vi "仪器参数设置.vi"(11 "仪器参数":T1) -> (2 "仪器参数 2":T1, 3 "check？":bool)   [LabVIEW 2016, in "斯坦道总磷.lvlib"]
uses:
  <vilib>/Utility/miscctls.llb/LVPointTypeDef.ctl
  <vilib>/addons/database/Auxilliary.llb/DB Tools DataTypes.ctl
  <vilib>/regexp/Match Regular Expression.xnode
  <vilib>/addons/database/NI_Database_API.lvlib
panel:
  in  "仪器参数表":i32(listbox)
  in  "取消":bool
  in  "确定":bool
  # "仪器参数"
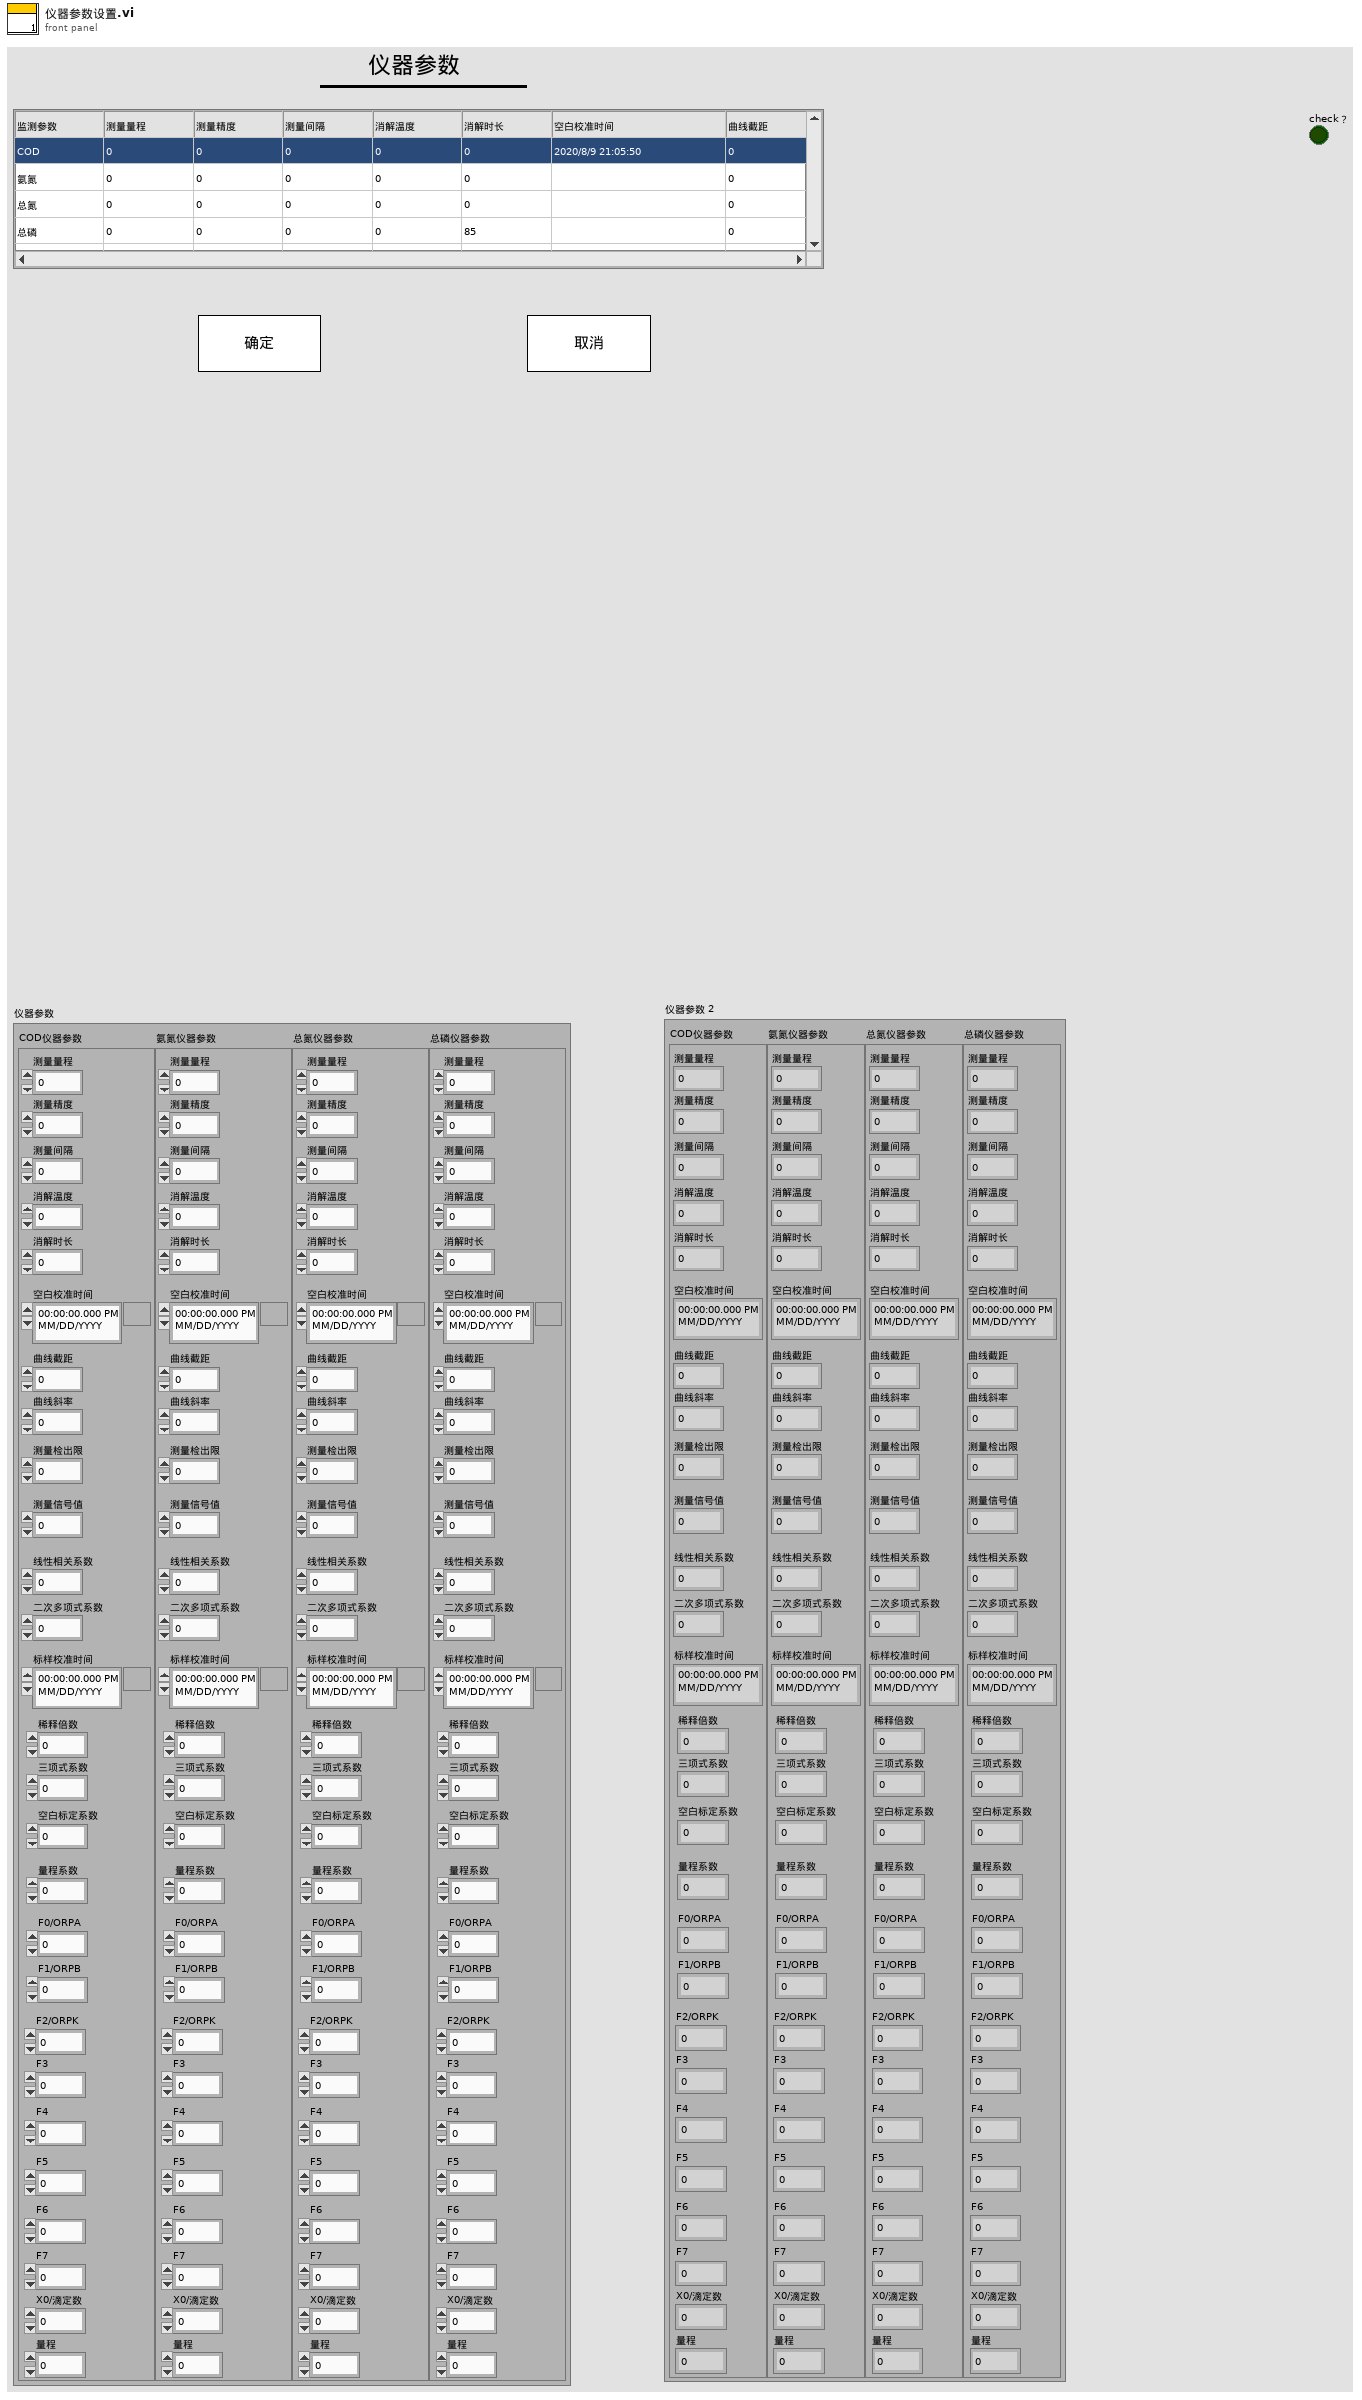
[diagram p1: front panel]
types:
  T1 = cluster{"COD仪器参数":cluster{"测量量程":dbl, "测量精度":dbl, "测量间隔":dbl, "消解温度":dbl, "消解时长":dbl, "空白校准时间":timestamp, "曲线截距":dbl, "曲线斜率":dbl, "测量检出限":dbl, "测量信号值":dbl, "线性相关系数":dbl, "二次多项式系数":dbl, "标样校准时间":timestamp, "稀释倍数":dbl, "三项式系数":dbl, "空白标定系数":dbl, "量程系数":dbl, "F0/ORPA":dbl, "F1/ORPB":dbl, "F2/ORPK":dbl, "F3":dbl, "F4":dbl, "F5":dbl, "F6":dbl, "F7":dbl, "X0/滴定数":dbl, "量程":dbl}, "氨氮仪器参数":cluster{"测量量程":dbl, "测量精度":dbl, "测量间隔":dbl, "消解温度":dbl, "消解时长":dbl, "空白校准时间":timestamp, "曲线截距":dbl, "曲线斜率":dbl, "测量检出限":dbl, "测量信号值":dbl, "线性相关系数":dbl, "二次多项式系数":dbl, "标样校准时间":timestamp, "稀释倍数":dbl, "三项式系数":dbl, "空白标定系数":dbl, "量程系数":dbl, "F0/ORPA":dbl, "F1/ORPB":dbl, "F2/ORPK":dbl, "F3":dbl, "F4":dbl, "F5":dbl, "F6":dbl, "F7":dbl, "X0/滴定数":dbl, "量程":dbl}, "总氮仪器参数":cluster{"测量量程":dbl, "测量精度":dbl, "测量间隔":dbl, "消解温度":dbl, "消解时长":dbl, "空白校准时间":timestamp, "曲线截距":dbl, "曲线斜率":dbl, "测量检出限":dbl, "测量信号值":dbl, "线性相关系数":dbl, "二次多项式系数":dbl, "标样校准时间":timestamp, "稀释倍数":dbl, "三项式系数":dbl, "空白标定系数":dbl, "量程系数":dbl, "F0/ORPA":dbl, "F1/ORPB":dbl, "F2/ORPK":dbl, "F3":dbl, "F4":dbl, "F5":dbl, "F6":dbl, "F7":dbl, "X0/滴定数":dbl, "量程":dbl}, "总磷仪器参数":cluster{"测量量程":dbl, "测量精度":dbl, "测量间隔":dbl, "消解温度":dbl, "消解时长":dbl, "空白校准时间":timestamp, "曲线截距":dbl, "曲线斜率":dbl, "测量检出限":dbl, "测量信号值":dbl, "线性相关系数":dbl, "二次多项式系数":dbl, "标样校准时间":timestamp, "稀释倍数":dbl, "三项式系数":dbl, "空白标定系数":dbl, "量程系数":dbl, "F0/ORPA":dbl, "F1/ORPB":dbl, "F2/ORPK":dbl, "F3":dbl, "F4":dbl, "F5":dbl, "F6":dbl, "F7":dbl, "X0/滴定数":dbl, "量程":dbl}}
  T2 = typedef "NI_Database_API.lvlib/DB Tools DataTypes.ctl" = enum16{"String", "Long (I32)", "Single (SGL)", "Double (DBL)", "Date/Time", "Binary"}
  T3 = typedef "LVPointTypeDef.ctl" = cluster{"Horizontal":i16, "Vertical":i16}
  T4 = typedef "LVPoint32TypeDef.ctl" = cluster{"Horizontal":i32, "Vertical":i32}
  T5 = typedef "LVRowAndColumnTypeDef.ctl" = cluster{"Row":i32, "Column":i32}
  T6 = cluster{"COD":bool, "氨氮":bool, "总氮":bool, "总磷":bool}
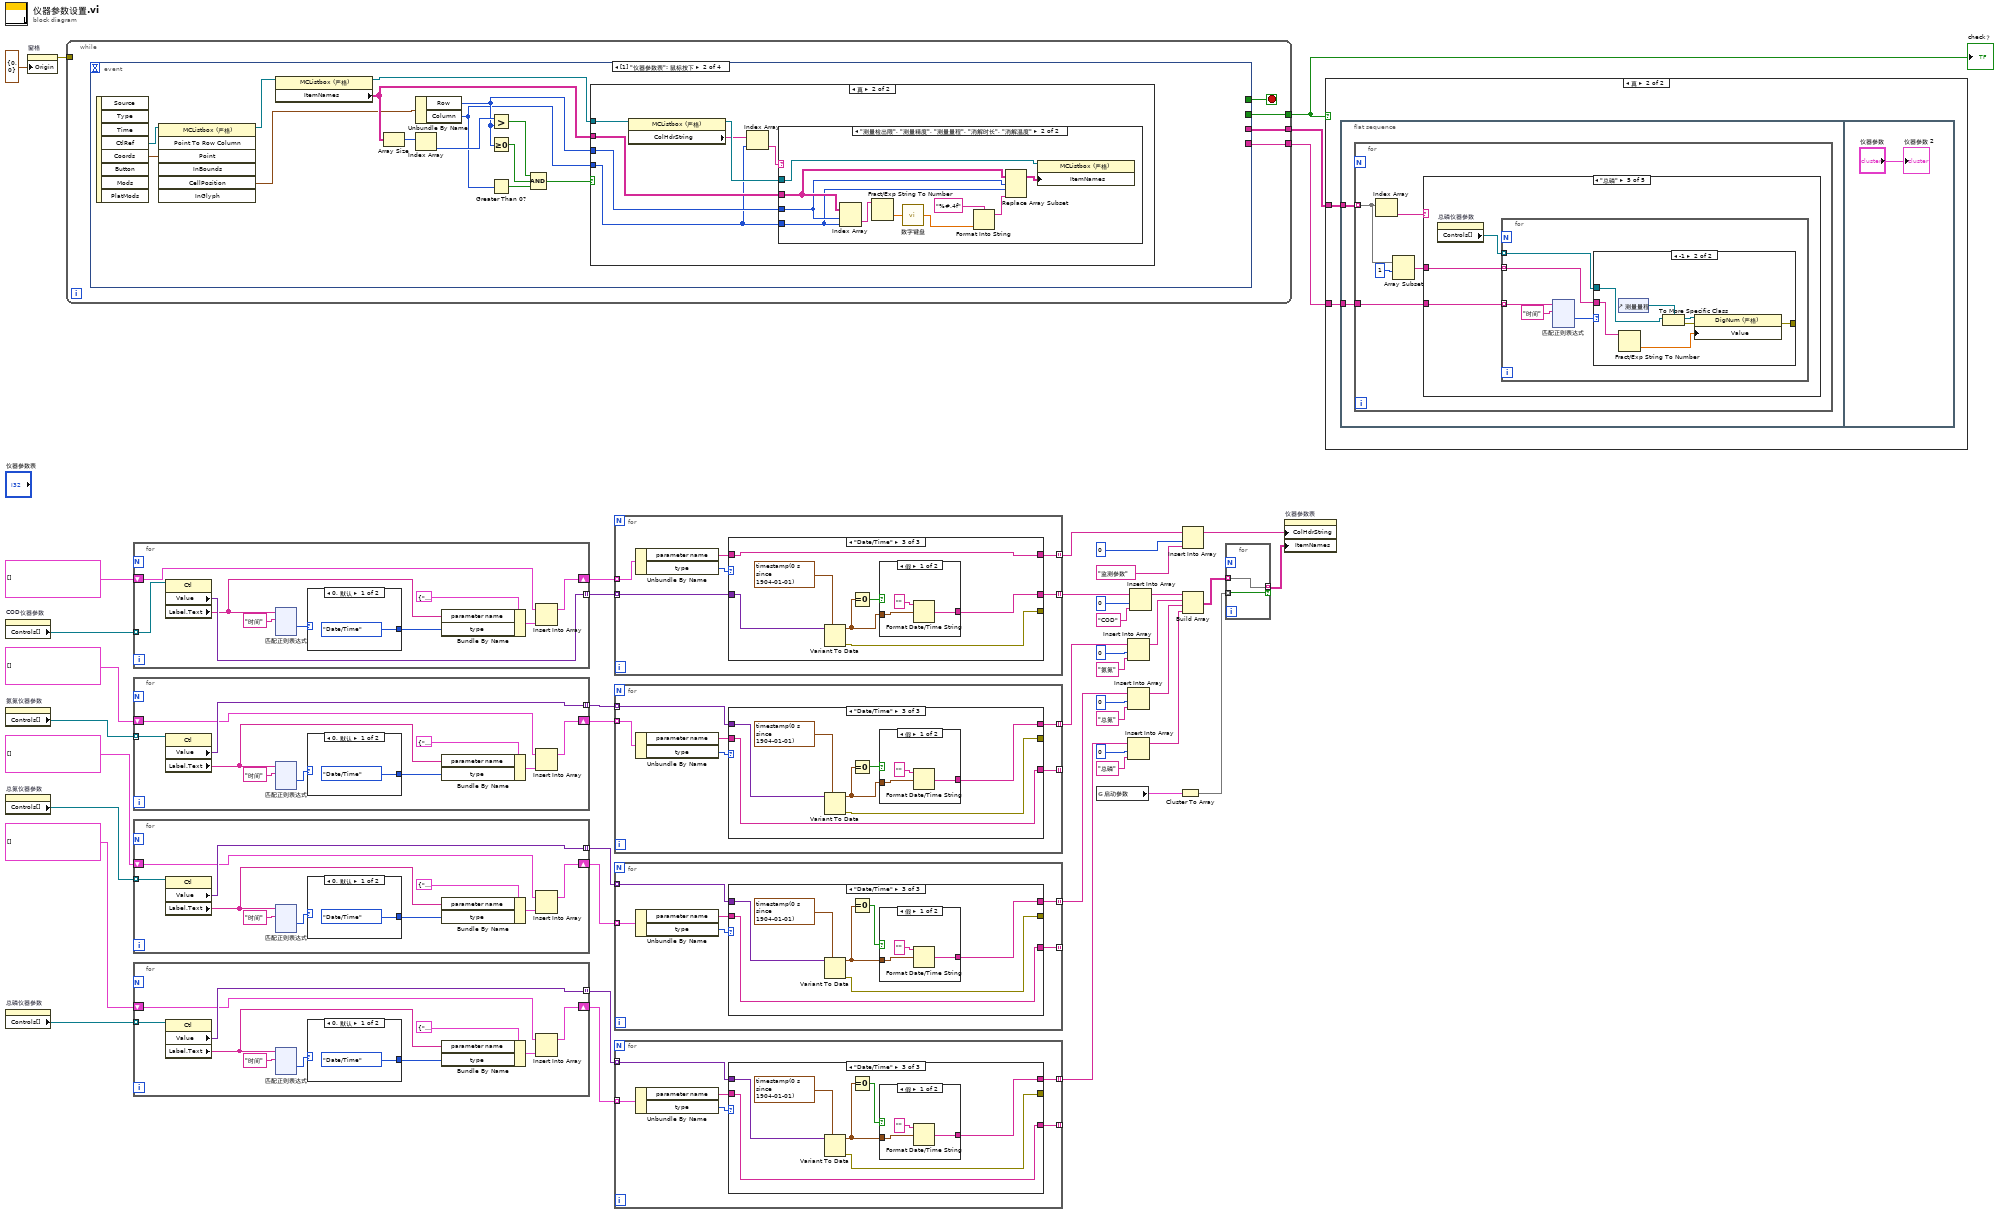
[diagram p0: block diagram]
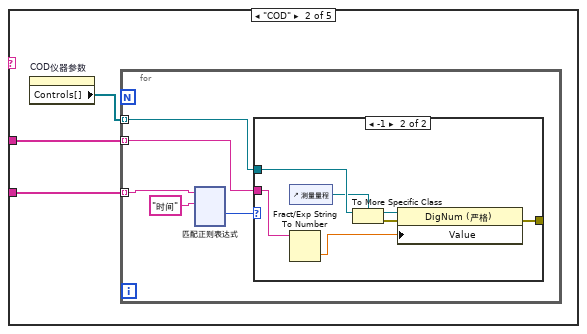
[diagram p4: hidden frame]
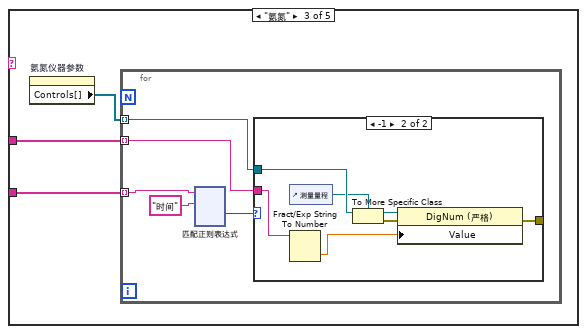
[diagram p6: hidden frame]
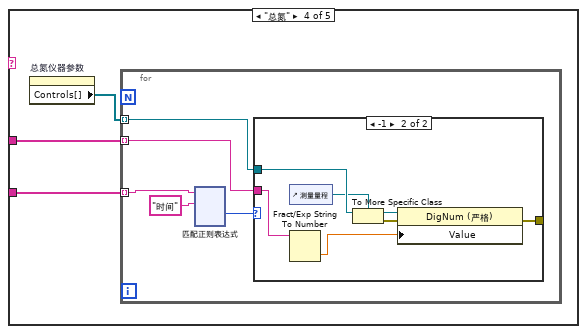
[diagram p8: hidden frame]
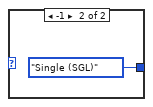
[diagram p11: hidden frame]
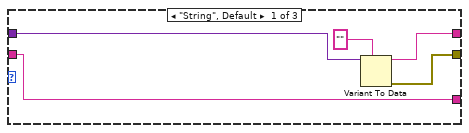
[diagram p12: hidden frame]
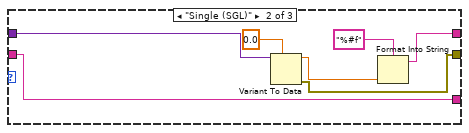
[diagram p13: hidden frame]
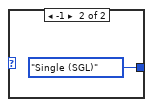
[diagram p15: hidden frame]
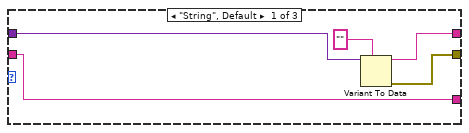
[diagram p16: hidden frame]
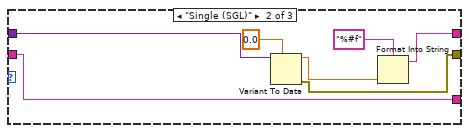
[diagram p17: hidden frame]
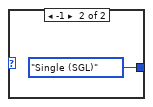
[diagram p19: hidden frame]
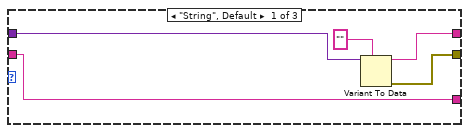
[diagram p20: hidden frame]
diagram:
  n1 = property on="COD仪器参数" class="Clust (严格)"() -> ("Controls[]"=w39:refnum<vi>[])  [unwired: 2 in, 2 out]
  n2 = property on="氨氮仪器参数" class="Clust (严格)"() -> ("Controls[]"=w38:refnum<vi>[])  [unwired: 2 in, 2 out]
  n3 = property on="总氮仪器参数" class="Clust (严格)"() -> ("Controls[]"=w31:refnum<vi>[])  [unwired: 2 in, 2 out]
  n4 = property on="总磷仪器参数" class="Clust (严格)"() -> ("Controls[]"=w30:refnum<vi>[])  [unwired: 2 in, 2 out]
  n5 = property on="窗格" class="Pane"("Origin"=T3 {"Horizontal"=0, "Vertical"=0} ("原点")) -> (error out=w44:errorcluster)  [unwired: 2 in, 1 out]
  n6 = while {
    tunnel: w44 -> [_]
    tunnel: [w48] -> w7
    tunnel: [w47] -> w6
    tunnel: [w46] -> w5
    stop <- w49 stop-if-true
    n7 = event shown="[1] \"仪器参数表\": 鼠标按下" {
      selector: _ -> [_ _ _ _]
      dyn-events: _ -> [_ _ _ _]
      timeout: _ -> [_ _ _ _]
      tunnel: [_ _ TRUE TRUE] -> w49
      tunnel: [_ _ _ "确定"] -> w48
      tunnel: [_ _ _ w83] -> w47
      tunnel: [_ _ _ w82] -> w46
      event Timeout {
        n8 = event-data() -> ()  [unwired: 1 in, 3 out]
      }
      event "仪器参数表": Mouse Down {
        n9 = event-data() -> ("CtlRef"=w63:refnum<vi>, "Coords"=w62:T4)  [unwired: 1 in, 6 out]
        n10 = invoke class="MCListbox (严格)" method="Point To Row Column"(reference=w63, "Point"=w62) -> (reference out=w51:refnum<vi>, "CellPosition"=w50:T5)  [unwired: 5 in, 5 out]
        n11 = property class="MCListbox (严格)"(reference=w51) -> (reference out=w52:refnum<vi>, "ItemNames"=w55:string[][])  [unwired: 1 in, 1 out]
        n12 = Array Size(array=w55) -> (size(s)=w59:i32[])
        n13 = Unbundle By Name(w50) -> ("Row"=w54:i32, "Column"=w53:i32)
        n14 = Index Array(array=w59) -> (element=w58:i32)  [unwired: 1 in]
        n15 = Greater?(x=w58, y=w54) -> (0:w57:bool)
        n16 = Greater Or Equal To 0?(x=w54) -> (x >= 0?=w56:bool)
        n17 = Greater Than 0?(x=w53) -> (x > 0?=w61:bool)
        n18 = Compound Arithmetic op=AND ("复合运算")(w57, w56, w61) -> (w60:bool)
        n19 = case shown="真" w60 {
          tunnel: w55 -> [_ w70]
          tunnel: w54 -> [_ w69]
          tunnel: w53 -> [_ w65]
          tunnel: w52 -> [_ w68]
          frame False {
          }
          frame True {
            n20 = property class="MCListbox (严格)"(reference=w68) -> (reference out=w67:refnum<vi>, "ColHdrString"=w66:string[])  [unwired: 1 in, 1 out]
            n21 = Index Array(array=w66, index=w65) -> (element=w64:string)
            n22 = case shown="\"测量检出限\", \"测量精度\", \"测量量程\", \"消解时长\", \"消解温度\"" w64 {
              tunnel: w70 -> [_ w76]
              tunnel: w69 -> [_ w75]
              tunnel: w65 -> [_ w74]
              tunnel: w67 -> [_ w71]
              frame Default {
              }
              frame "测量检出限", "测量精度", "测量量程", "消解时长", "消解温度" {
                n23 = Index Array(array=w76, index (row)=w75, index (col)=w74) -> (element=w80:string)
                n24 = Fract/Exp String To Number(string=w80) -> (number=w79:dbl)  [unwired: 3 in, 1 out]
                n25 = call "数字键盘.vi"("OldNumber"=w79) -> ("NewNumber"=w78:dbl)
                n26 = Format Into String(format string="%#.4f" ("格式字符串"), w78) -> (resulting string=w73:string)  [unwired: 2 in, 1 out]
                n27 = Replace Array Subset(array=w76, new element=w73, index (row)=w75, index (col)=w74) -> (w72:string[][])
                n28 = property class="MCListbox (严格)"(reference=w71, "ItemNames"=w72) -> ()  [unwired: 1 in, 2 out]
              }
            }
          }
        }
      }
      event "取消": Value Change; Panel Close {
        n29 = event-data() -> ()  [unwired: 1 in, 3 out]
      }
      event "确定": Value Change {
        n30 = event-data() -> ()  [unwired: 1 in, 6 out]
        n31 = property on="仪器参数表" class="MCListbox (严格)"() -> ("ItemNames"=w83:string[][], "ColHdrString"=w82:string[])  [unwired: 2 in, 2 out]
      }
    }
  }
  "check？" <- w7
  n32 = for {
    tunnel: w39 -> [w95] mode=indexing
    tunnel: [w94] -> w43 mode=indexing
    shift-right: [w92] -> w40
    shift-left: cluster{"parameter name":string, "type":T2}[] [] ("parameters out") -> [w93]
    n33 = property class="Ctl"(reference=w95) -> ("Value"=w94:variant, "Label.Text"=w90:string)  [unwired: 1 in, 2 out]
    n34 = xnode "匹配正则表达式"("输入字符串"=w90, "正则表达式"="时间") -> ("匹配后偏移量"=w88:i32)  [unwired: 4 in, 4 out]
    n35 = case shown="0, 默认" w88 {
      tunnel: [DB_Tools_DataTypes."Date/Time" ("type") DB_Tools_DataTypes."Single (SGL)" ("type")] -> w87
      frame 0, Default {
      }
      frame -1 {
      }
    }
    n36 = Bundle By Name(cluster=cluster{"parameter name":string, "type":T2} {"parameter name"="", "type"=enum."String"} ("parameter information"), "parameter name"=w90, "type"=w87) -> (w86:cluster{"parameter name":string, "type":T2})
    n37 = Insert Into Array(array=w93, new element=w86) -> (w92:cluster{"parameter name":string, "type":T2}[])  [unwired: 1 in]
  }
  n38 = for {
    tunnel: w38 -> [w221] mode=indexing
    tunnel: [w220] -> w35 mode=indexing
    shift-right: [w218] -> w37
    shift-left: cluster{"parameter name":string, "type":T2}[] [] ("parameters out") -> [w219]
    n39 = property class="Ctl"(reference=w221) -> ("Value"=w220:variant, "Label.Text"=w216:string)  [unwired: 1 in, 2 out]
    n40 = xnode "匹配正则表达式"("输入字符串"=w216, "正则表达式"="时间") -> ("匹配后偏移量"=w214:i32)  [unwired: 4 in, 4 out]
    n41 = case shown="0, 默认" w214 {
      tunnel: [DB_Tools_DataTypes."Date/Time" ("type") DB_Tools_DataTypes."Single (SGL)" ("type")] -> w213
      frame 0, Default {
      }
      frame -1 {
      }
    }
    n42 = Bundle By Name(cluster=cluster{"parameter name":string, "type":T2} {"parameter name"="", "type"=enum."String"} ("parameter information"), "parameter name"=w216, "type"=w213) -> (w212:cluster{"parameter name":string, "type":T2})
    n43 = Insert Into Array(array=w219, new element=w212) -> (w218:cluster{"parameter name":string, "type":T2}[])  [unwired: 1 in]
  }
  n44 = for {
    tunnel: w31 -> [w347] mode=indexing
    tunnel: [w346] -> w34 mode=indexing
    shift-right: [w344] -> w32
    shift-left: cluster{"parameter name":string, "type":T2}[] [] ("parameters out") -> [w345]
    n45 = property class="Ctl"(reference=w347) -> ("Value"=w346:variant, "Label.Text"=w342:string)  [unwired: 1 in, 2 out]
    n46 = xnode "匹配正则表达式"("输入字符串"=w342, "正则表达式"="时间") -> ("匹配后偏移量"=w340:i32)  [unwired: 4 in, 4 out]
    n47 = case shown="0, 默认" w340 {
      tunnel: [DB_Tools_DataTypes."Date/Time" ("type") DB_Tools_DataTypes."Single (SGL)" ("type")] -> w339
      frame 0, Default {
      }
      frame -1 {
      }
    }
    n48 = Bundle By Name(cluster=cluster{"parameter name":string, "type":T2} {"parameter name"="", "type"=enum."String"} ("parameter information"), "parameter name"=w342, "type"=w339) -> (w338:cluster{"parameter name":string, "type":T2})
    n49 = Insert Into Array(array=w345, new element=w338) -> (w344:cluster{"parameter name":string, "type":T2}[])  [unwired: 1 in]
  }
  n50 = for {
    tunnel: w30 -> [w473] mode=indexing
    tunnel: [w472] -> w27 mode=indexing
    shift-right: [w470] -> w29
    shift-left: cluster{"parameter name":string, "type":T2}[] [] ("parameters out") -> [w471]
    n51 = property class="Ctl"(reference=w473) -> ("Value"=w472:variant, "Label.Text"=w468:string)  [unwired: 1 in, 2 out]
    n52 = xnode "匹配正则表达式"("输入字符串"=w468, "正则表达式"="时间") -> ("匹配后偏移量"=w466:i32)  [unwired: 4 in, 4 out]
    n53 = case shown="0, 默认" w466 {
      tunnel: [DB_Tools_DataTypes."Date/Time" ("type") DB_Tools_DataTypes."Single (SGL)" ("type")] -> w465
      frame 0, Default {
      }
      frame -1 {
      }
    }
    n54 = Bundle By Name(cluster=cluster{"parameter name":string, "type":T2} {"parameter name"="", "type"=enum."String"} ("parameter information"), "parameter name"=w468, "type"=w465) -> (w464:cluster{"parameter name":string, "type":T2})
    n55 = Insert Into Array(array=w471, new element=w464) -> (w470:cluster{"parameter name":string, "type":T2}[])  [unwired: 1 in]
  }
  n56 = for {
    tunnel: w40 -> [w595] mode=indexing
    tunnel: w43 -> [w593] mode=indexing
    tunnel: [w591] -> w41 mode=indexing
    tunnel: [w590] -> w23 mode=indexing
    n57 = Unbundle By Name(w595) -> ("parameter name"=w592:string, "type"=w594:T2)
    n58 = case shown="\"Date/Time\"" w594 {
      tunnel: w593 -> [w599 w607 w614]
      tunnel: w592 -> [w598 w606 w612]
      tunnel: [w598 w606 w612] -> w591
      tunnel: [w597 w601 w610] -> w590
      tunnel: [w596 w605 w611] -> _
      frame "String", Default {
        n59 = Variant To Data(type="", Variant=w599) -> (data=w597:string, error out=w596:errorcluster)  [unwired: 1 in]
      }
      frame "Single (SGL)" {
        n60 = Variant To Data(type=sgl 0.0, Variant=w607) -> (data=w603:sgl, error out=w605:errorcluster)  [unwired: 1 in]
        n61 = Format Into String(format string="%#f" ("格式字符串"), w603) -> (resulting string=w601:string)  [unwired: 2 in, 1 out]
      }
      frame "Date/Time" {
        n62 = Variant To Data(type=timestamp(0 s since 1904-01-01) ("时间标识"), Variant=w614) -> (data=w609:timestamp, error out=w611:errorcluster)  [unwired: 1 in]
        n63 = Equal To 0?(x=w609) -> (x = 0?=w608:bool)
        n64 = case shown="假" w608 {
          tunnel: [w617 _] -> w610
          tunnel: w609 -> [w615 _]
          frame False {
            n65 = Format Date/Time String(time format string (%c)="" ("时间格式字符串(%c)"), seconds (now)=w615) -> (date/time string=w617:string)  [unwired: 1 in]
          }
          frame True {
          }
        }
      }
    }
  }
  n66 = for {
    tunnel: w37 -> [w623] mode=indexing
    tunnel: w35 -> [w621] mode=indexing
    tunnel: [w619] -> _ mode=indexing
    tunnel: [w618] -> w14 mode=indexing
    n67 = Unbundle By Name(w623) -> ("parameter name"=w620:string, "type"=w622:T2)
    n68 = case shown="\"Date/Time\"" w622 {
      tunnel: w621 -> [w627 w635 w642]
      tunnel: w620 -> [w626 w634 w640]
      tunnel: [w626 w634 w640] -> w619
      tunnel: [w625 w629 w638] -> w618
      tunnel: [w624 w633 w639] -> _
      frame "String", Default {
        n69 = Variant To Data(type="", Variant=w627) -> (data=w625:string, error out=w624:errorcluster)  [unwired: 1 in]
      }
      frame "Single (SGL)" {
        n70 = Variant To Data(type=sgl 0.0, Variant=w635) -> (data=w631:sgl, error out=w633:errorcluster)  [unwired: 1 in]
        n71 = Format Into String(format string="%#f" ("格式字符串"), w631) -> (resulting string=w629:string)  [unwired: 2 in, 1 out]
      }
      frame "Date/Time" {
        n72 = Variant To Data(type=timestamp(0 s since 1904-01-01) ("时间标识"), Variant=w642) -> (data=w637:timestamp, error out=w639:errorcluster)  [unwired: 1 in]
        n73 = Equal To 0?(x=w637) -> (x = 0?=w636:bool)
        n74 = case shown="假" w636 {
          tunnel: [w645 _] -> w638
          tunnel: w637 -> [w643 _]
          frame False {
            n75 = Format Date/Time String(time format string (%c)="" ("时间格式字符串(%c)"), seconds (now)=w643) -> (date/time string=w645:string)  [unwired: 1 in]
          }
          frame True {
          }
        }
      }
    }
  }
  n76 = for {
    tunnel: w32 -> [w651] mode=indexing
    tunnel: w34 -> [w649] mode=indexing
    tunnel: [w647] -> _ mode=indexing
    tunnel: [w646] -> w13 mode=indexing
    n77 = Unbundle By Name(w651) -> ("parameter name"=w648:string, "type"=w650:T2)
    n78 = case shown="\"Date/Time\"" w650 {
      tunnel: w649 -> [w655 w663 w670]
      tunnel: w648 -> [w654 w662 w668]
      tunnel: [w654 w662 w668] -> w647
      tunnel: [w653 w657 w666] -> w646
      tunnel: [w652 w661 w667] -> _
      frame "String", Default {
        n79 = Variant To Data(type="", Variant=w655) -> (data=w653:string, error out=w652:errorcluster)  [unwired: 1 in]
      }
      frame "Single (SGL)" {
        n80 = Variant To Data(type=sgl 0.0, Variant=w663) -> (data=w659:sgl, error out=w661:errorcluster)  [unwired: 1 in]
        n81 = Format Into String(format string="%#f" ("格式字符串"), w659) -> (resulting string=w657:string)  [unwired: 2 in, 1 out]
      }
      frame "Date/Time" {
        n82 = Variant To Data(type=timestamp(0 s since 1904-01-01) ("时间标识"), Variant=w670) -> (data=w665:timestamp, error out=w667:errorcluster)  [unwired: 1 in]
        n83 = Equal To 0?(x=w665) -> (x = 0?=w664:bool)
        n84 = case shown="假" w664 {
          tunnel: w665 -> [w673 _]
          tunnel: [w672 _] -> w666
          frame False {
            n85 = Format Date/Time String(time format string (%c)="" ("时间格式字符串(%c)"), seconds (now)=w673) -> (date/time string=w672:string)  [unwired: 1 in]
          }
          frame True {
          }
        }
      }
    }
  }
  n86 = for {
    tunnel: w29 -> [w679] mode=indexing
    tunnel: w27 -> [w677] mode=indexing
    tunnel: [w675] -> _ mode=indexing
    tunnel: [w674] -> w12 mode=indexing
    n87 = Unbundle By Name(w679) -> ("parameter name"=w676:string, "type"=w678:T2)
    n88 = case shown="\"Date/Time\"" w678 {
      tunnel: w677 -> [w683 w691 w698]
      tunnel: w676 -> [w682 w690 w696]
      tunnel: [w682 w690 w696] -> w675
      tunnel: [w681 w685 w694] -> w674
      tunnel: [w680 w689 w695] -> _
      frame "String", Default {
        n89 = Variant To Data(type="", Variant=w683) -> (data=w681:string, error out=w680:errorcluster)  [unwired: 1 in]
      }
      frame "Single (SGL)" {
        n90 = Variant To Data(type=sgl 0.0, Variant=w691) -> (data=w687:sgl, error out=w689:errorcluster)  [unwired: 1 in]
        n91 = Format Into String(format string="%#f" ("格式字符串"), w687) -> (resulting string=w685:string)  [unwired: 2 in, 1 out]
      }
      frame "Date/Time" {
        n92 = Variant To Data(type=timestamp(0 s since 1904-01-01) ("时间标识"), Variant=w698) -> (data=w693:timestamp, error out=w695:errorcluster)  [unwired: 1 in]
        n93 = Equal To 0?(x=w693) -> (x = 0?=w692:bool)
        n94 = case shown="假" w692 {
          tunnel: w693 -> [w701 _]
          tunnel: [w700 _] -> w694
          frame False {
            n95 = Format Date/Time String(time format string (%c)="" ("时间格式字符串(%c)"), seconds (now)=w701) -> (date/time string=w700:string)  [unwired: 1 in]
          }
          frame True {
          }
        }
      }
    }
  }
  n96 = global read "总磷总氮断电保存全局变量.vi" "启动参数"() -> (w4:T6)
  n97 = Insert Into Array(array=w14, index=0 ("索引"), new element="氨氮" ("新元素/子数组")) -> (w10:string[])
  n98 = Insert Into Array(array=w13, index=0 ("索引"), new element="总氮" ("新元素/子数组")) -> (w9:string[])
  n99 = Insert Into Array(array=w12, index=0 ("索引"), new element="总磷" ("新元素/子数组")) -> (w8:string[])
  n100 = Insert Into Array(array=w23, index=0 ("索引"), new element="COD" ("新元素/子数组")) -> (w11:string[])
  n101 = Cluster To Array(cluster=w4) -> (array=w3:bool[])
  n102 = Insert Into Array(array=w41, index=0 ("索引"), new element="监测参数" ("新元素/子数组")) -> (w26:string[])
  n103 = Build Array(w11, w10, w9, w8) -> (w2:string[][])
  n104 = for {
    tunnel: w3 -> [w702] mode=indexing
    tunnel: w2 -> [w703] mode=indexing
    tunnel: [w703] -> w1 mode=indexing if=w702
  }
  n105 = property on="仪器参数表" class="MCListbox (严格)"("ColHdrString"=w26, "ItemNames"=w1) -> ()  [unwired: 2 in, 2 out]
  n106 = case shown="真" w7 {
    tunnel: w6 -> [_ w705]
    tunnel: w5 -> [_ w704]
    frame False {
    }
    frame True {
      n107 = flat-sequence {
        tunnel: w705 -> [w707]
        tunnel: w704 -> [w706]
        frame #0 {
          n108 = for {
            tunnel: w707 -> [w711] mode=indexing
            tunnel: w706 -> [w708]
            n109 = Index Array(array=w711) -> (element=w712:string)  [unwired: 1 in]
            n110 = Array Subset(array=w711, index=1 ("索引")) -> (w709:string[])  [unwired: 1 in]
            n111 = case shown="\"总磷\"" w712 {
              tunnel: w709 -> [_ w715 w844 w973 w1102]
              tunnel: w708 -> [_ w714 w843 w972 w1101]
              frame Default {
              }
              frame "COD" {
                n112 = property on="COD仪器参数" class="Clust (严格)"() -> ("Controls[]"=w713:refnum<vi>[])  [unwired: 2 in, 2 out]
                n113 = for {
                  tunnel: w715 -> [w716] mode=indexing
                  tunnel: w714 -> [w720] mode=indexing
                  tunnel: w713 -> [w717] mode=indexing
                  n114 = xnode "匹配正则表达式"("输入字符串"=w720, "正则表达式"="时间") -> ("匹配后偏移量"=w718:i32)  [unwired: 4 in, 4 out]
                  n115 = case shown="-1" w718 {
                    tunnel: w717 -> [_ w727]
                    tunnel: w716 -> [_ w724]
                    tunnel: [_ w721] -> _
                    frame 0, Default {
                    }
                    frame -1 {
                      n116 = control-ref of="测量量程"() -> (w725:refnum<vi>)
                      n117 = Fract/Exp String To Number(string=w724) -> (number=w723:dbl)  [unwired: 3 in, 1 out]
                      n118 = To More Specific Class(target class=w725, reference=w727) -> (specific class reference=w726:refnum<vi>, error out=w722:errorcluster)  [unwired: 1 in]
                      n119 = property class="DigNum (严格)"(reference=w726, error in=w722, "Value"=w723) -> (error out=w721:errorcluster)  [unwired: 1 out]
                    }
                  }
                }
              }
              frame "氨氮" {
                n120 = property on="氨氮仪器参数" class="Clust (严格)"() -> ("Controls[]"=w842:refnum<vi>[])  [unwired: 2 in, 2 out]
                n121 = for {
                  tunnel: w844 -> [w845] mode=indexing
                  tunnel: w843 -> [w849] mode=indexing
                  tunnel: w842 -> [w846] mode=indexing
                  n122 = xnode "匹配正则表达式"("输入字符串"=w849, "正则表达式"="时间") -> ("匹配后偏移量"=w847:i32)  [unwired: 4 in, 4 out]
                  n123 = case shown="-1" w847 {
                    tunnel: w846 -> [_ w856]
                    tunnel: w845 -> [_ w853]
                    tunnel: [_ w850] -> _
                    frame 0, Default {
                    }
                    frame -1 {
                      n124 = control-ref of="测量量程"() -> (w854:refnum<vi>)
                      n125 = Fract/Exp String To Number(string=w853) -> (number=w852:dbl)  [unwired: 3 in, 1 out]
                      n126 = To More Specific Class(target class=w854, reference=w856) -> (specific class reference=w855:refnum<vi>, error out=w851:errorcluster)  [unwired: 1 in]
                      n127 = property class="DigNum (严格)"(reference=w855, error in=w851, "Value"=w852) -> (error out=w850:errorcluster)  [unwired: 1 out]
                    }
                  }
                }
              }
              frame "总氮" {
                n128 = property on="总氮仪器参数" class="Clust (严格)"() -> ("Controls[]"=w971:refnum<vi>[])  [unwired: 2 in, 2 out]
                n129 = for {
                  tunnel: w973 -> [w974] mode=indexing
                  tunnel: w972 -> [w978] mode=indexing
                  tunnel: w971 -> [w975] mode=indexing
                  n130 = xnode "匹配正则表达式"("输入字符串"=w978, "正则表达式"="时间") -> ("匹配后偏移量"=w976:i32)  [unwired: 4 in, 4 out]
                  n131 = case shown="-1" w976 {
                    tunnel: w975 -> [_ w985]
                    tunnel: w974 -> [_ w982]
                    tunnel: [_ w979] -> _
                    frame 0, Default {
                    }
                    frame -1 {
                      n132 = control-ref of="测量量程"() -> (w983:refnum<vi>)
                      n133 = Fract/Exp String To Number(string=w982) -> (number=w981:dbl)  [unwired: 3 in, 1 out]
                      n134 = To More Specific Class(target class=w983, reference=w985) -> (specific class reference=w984:refnum<vi>, error out=w980:errorcluster)  [unwired: 1 in]
                      n135 = property class="DigNum (严格)"(reference=w984, error in=w980, "Value"=w981) -> (error out=w979:errorcluster)  [unwired: 1 out]
                    }
                  }
                }
              }
              frame "总磷" {
                n136 = property on="总磷仪器参数" class="Clust (严格)"() -> ("Controls[]"=w1100:refnum<vi>[])  [unwired: 2 in, 2 out]
                n137 = for {
                  tunnel: w1102 -> [w1103] mode=indexing
                  tunnel: w1101 -> [w1107] mode=indexing
                  tunnel: w1100 -> [w1104] mode=indexing
                  n138 = xnode "匹配正则表达式"("输入字符串"=w1107, "正则表达式"="时间") -> ("匹配后偏移量"=w1105:i32)  [unwired: 4 in, 4 out]
                  n139 = case shown="-1" w1105 {
                    tunnel: w1104 -> [_ w1114]
                    tunnel: w1103 -> [_ w1111]
                    tunnel: [_ w1108] -> _
                    frame 0, Default {
                    }
                    frame -1 {
                      n140 = control-ref of="测量量程"() -> (w1112:refnum<vi>)
                      n141 = Fract/Exp String To Number(string=w1111) -> (number=w1110:dbl)  [unwired: 3 in, 1 out]
                      n142 = To More Specific Class(target class=w1112, reference=w1114) -> (specific class reference=w1113:refnum<vi>, error out=w1109:errorcluster)  [unwired: 1 in]
                      n143 = property class="DigNum (严格)"(reference=w1113, error in=w1109, "Value"=w1110) -> (error out=w1108:errorcluster)  [unwired: 1 out]
                    }
                  }
                }
              }
            }
          }
        }
        frame #1 {
          "仪器参数 2" <- "仪器参数"
        }
      }
    }
  }
